vi "from data to rad.vi"(1 "Radians low in":i32 caption="Degrees in", 2 "Radians high in":i32 caption="Degrees in") -> (0 "Radians":sgl)   [LabVIEW 2013]
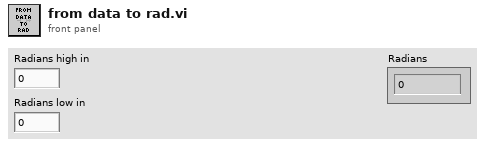
[diagram p1: front panel]
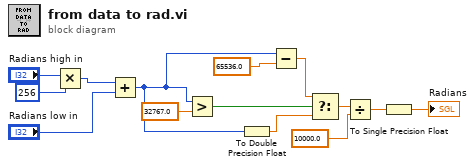
[diagram p0: block diagram]
diagram:
  n1 = Multiply(x="Radians high in", y=256) -> (x*y=w3:i32)
  n2 = Add(x=w3, y="Radians low in") -> (x+y=w1:i32)
  n3 = Greater?(x=w1, y=32767.0) -> (0:w13:bool)
  n4 = To Double Precision Float(number=w1) -> (double precision float=w9:dbl)
  n5 = Subtract(x=w1, y=65536.0) -> (x-y=w11:dbl)
  n6 = Select(t=w11, s=w13, f=w9) -> (s? t:f=w8:dbl)
  n7 = Divide(x=w8, y=10000.0) -> (x/y=w6:dbl)
  n8 = To Single Precision Float(number=w6) -> (single precision float=→"Radians":sgl)
